vi "Login (sub vi).vi"() -> (2 "Player\nname 2":string)   [LabVIEW 2014]
panel:
  in  "Player\nname":string
  in  "OK Button":bool
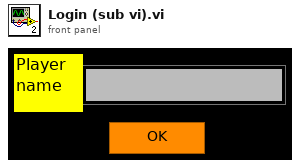
[diagram p1: front panel]
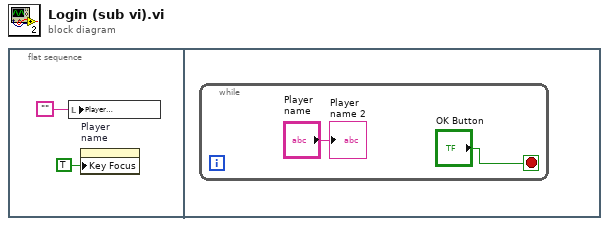
[diagram p0: block diagram]
diagram:
  n1 = flat-sequence {
    frame #0 {
      n2 = local write "Player\nname"("") -> ()
      n3 = property on="Player\nname" class="Str"("Key Focus"=TRUE) -> ()  [unwired: 2 in, 2 out]
    }
    frame #1 {
      n4 = while {
        stop <- "OK Button" stop-if-true
        "Player\nname 2" <- "Player\nname"
      }
    }
  }
